vi "parse key value pair.vi"(8 "error in (no error)":errorcluster, 11 "key value pair in":string) -> (0 "error out":errorcluster, 3 "key value pair out":T1)   [LabVIEW 2024, in "controls manager.lvlib"]
uses:
  controls manager.lvlib
  key value pair.ctl
  <vilib>/Utility/error.llb/Trim Whitespace One-Sided.vi
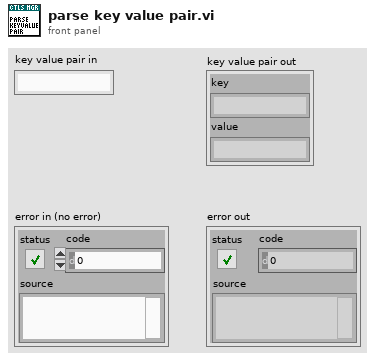
[diagram p1: front panel]
types:
  T1 = typedef "controls manager.lvlib/key value pair.ctl" = cluster{"key":string, "value":string}
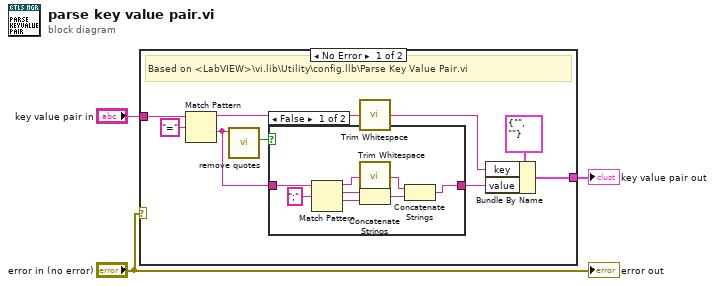
[diagram p0: block diagram]
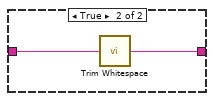
[diagram p2: hidden frame]
diagram:
  n1 = case shown="No Error" "error in (no error)" {
    tunnel: "key value pair in" -> [w11 _]
    tunnel: [w4 _] -> w1
    frame No Error {
      # "Based on <LabVIEW>\\vi.lib\\Utility\\config.llb\\Parse Key Value Pair.vi"
      n2 = Match Pattern(string=w11, regular expression="=") -> (before substring=w10:string, after substring=w8:string)  [unwired: 1 in, 2 out]
      n3 = call "remove quotes.vi"("string"=w8) -> ("in quotes?"=w9:bool)  [unwired: 8 in, 2 out]
      n4 = case shown="False" w9 {
        tunnel: [w13 w22] -> w5
        tunnel: w8 -> [w17 w21]
        frame False {
          n5 = Match Pattern(string=w17, regular expression=";") -> (before substring=w14:string, match substring=w19:string, after substring=w20:string)  [unwired: 1 in, 1 out]
          n6 = call <vilib>:"Trim Whitespace.vi"("string"=w14) -> ("trimmed string"=w15:string)  [unwired: 1 in]
          n7 = Concatenate Strings(w19, w20) -> (w16:string)
          n8 = Concatenate Strings(w15, w16) -> (w13:string)
        }
        frame True {
          n9 = call <vilib>:"Trim Whitespace.vi"("string"=w21) -> ("trimmed string"=w22:string)  [unwired: 1 in]
        }
      }
      n10 = call <vilib>:"Trim Whitespace.vi"("string"=w10) -> ("trimmed string"=w6:string)  [unwired: 1 in]
      n11 = Bundle By Name(cluster=T1 {"key"="", "value"=""}, "key"=w6, "value"=w5) -> (w4:T1)
    }
    frame Error {
    }
  }
  "key value pair out" <- w1
  "error out" <- "error in (no error)"
